vi "运行间隔计算.vi"(11 "运行周期":i16=4) -> (3 "数组":i32[](array[numeric]))   [LabVIEW 2016, in "PLC.lvlib"]
uses:
  PLC.lvlib
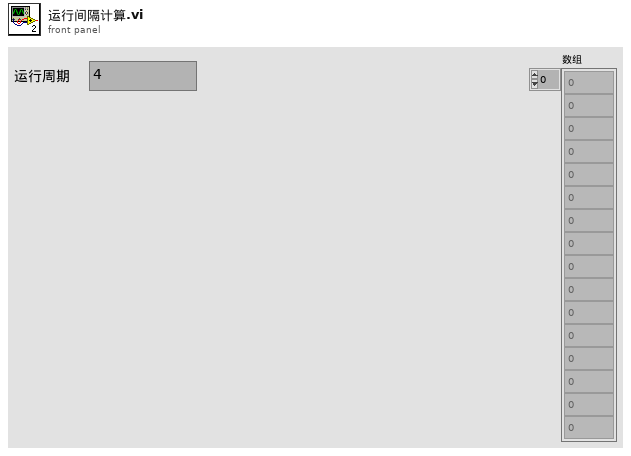
[diagram p1: front panel]
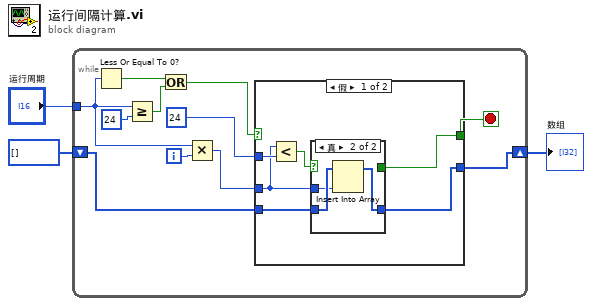
[diagram p0: block diagram]
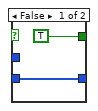
[diagram p2: hidden frame]
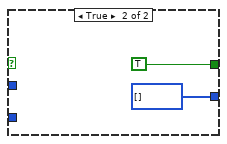
[diagram p3: hidden frame]
diagram:
  n1 = while {
    tunnel: "运行周期" -> [w8]
    shift-right: [w12] -> w1
    shift-left: i32[] [] -> [w13]
    i -> [w14]
    stop <- w10 stop-if-true
    n2 = Less Or Equal To 0?(x=w8) -> (x <= 0?=w5:bool)
    n3 = Greater Or Equal?(x=w8, y=i16 24) -> (x >= y?=w6:bool)
    n4 = Or(x=w5, y=w6) -> (x .or. y?=w4:bool)
    n5 = Multiply(x=w8, y=w14) -> (x*y=w9:i32)
    n6 = case shown="假" w4 {
      tunnel: w13 -> [w20 _]
      tunnel: [w19 i32[] []] -> w12
      tunnel: 24 ("y") -> [w18 _]
      tunnel: [w16 TRUE] -> w10
      tunnel: w9 -> [w15 _]
      frame False {
        n7 = Less?(x=w15, y=w18) -> (x < y?=w17:bool)
        n8 = case shown="真" w17 {
          tunnel: w20 -> [w22 w25]
          tunnel: [w22 w24] -> w19
          tunnel: [TRUE _] -> w16
          tunnel: w15 -> [_ w23]
          frame False {
          }
          frame True {
            n9 = Insert Into Array(array=w25, new element=w23) -> (w24:i32[])  [unwired: 1 in]
          }
        }
      }
      frame True {
      }
    }
  }
  "数组" <- w1
